vi "DailyReportTry.vi"() -> ()   [LabVIEW 2012]
uses:
  <vilib>/addons/database/Auxilliary.llb/DB Tools Cursor Type.ctl
  <vilib>/addons/database/Connection.llb/DB Tools Open Connec (Path).vi
  <vilib>/addons/database/Connection.llb/Conn Execute.vi
  <vilib>/addons/database/Recordset.llb/Rec Fetch Recordset Data (R).vi
  <vilib>/addons/database/Recordset.llb/Rec Destroy - Connection.vi
  <vilib>/addons/database/_DB Variant To Data/Database Variant To Data.xnode
  <vilib>/addons/database/NI_Database_API.lvlib
panel:
  out "trimmed string":string
  in  "Customer":string(combo)
  in  "error in (no error)":errorcluster
  out "error out":errorcluster
  in  "input cluster":cluster{"String":string, "Value":string}
  in  "connection information":path=path "c:/m100/data/m1003.dsn"
  in  "Device":string(combo)
  out "Boolean":bool
  in  "From Date (起日)":string="2014/9/20"
  in  "離開":bool
  in  "執行":bool
  in  "Shift (班別)":string(combo)
  in  "End Date (ùら)":string="2014/9/24"
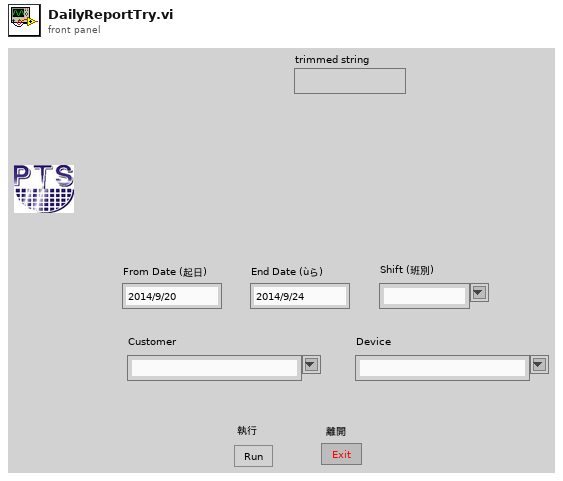
[diagram p1: front panel]
types:
  T1 = typedef "NI_Database_API.lvlib/DB Tools Cursor Type.ctl" = enum16{"forward-only", "keyset", "dynamic", "static"}
  T2 = typedef "NI_Database_API.lvlib/Conn ObjectReference.ctl" = refnum<k1>
  T3 = typedef "NI_Database_API.lvlib/Rec ObjectReference.ctl" = refnum<k1>
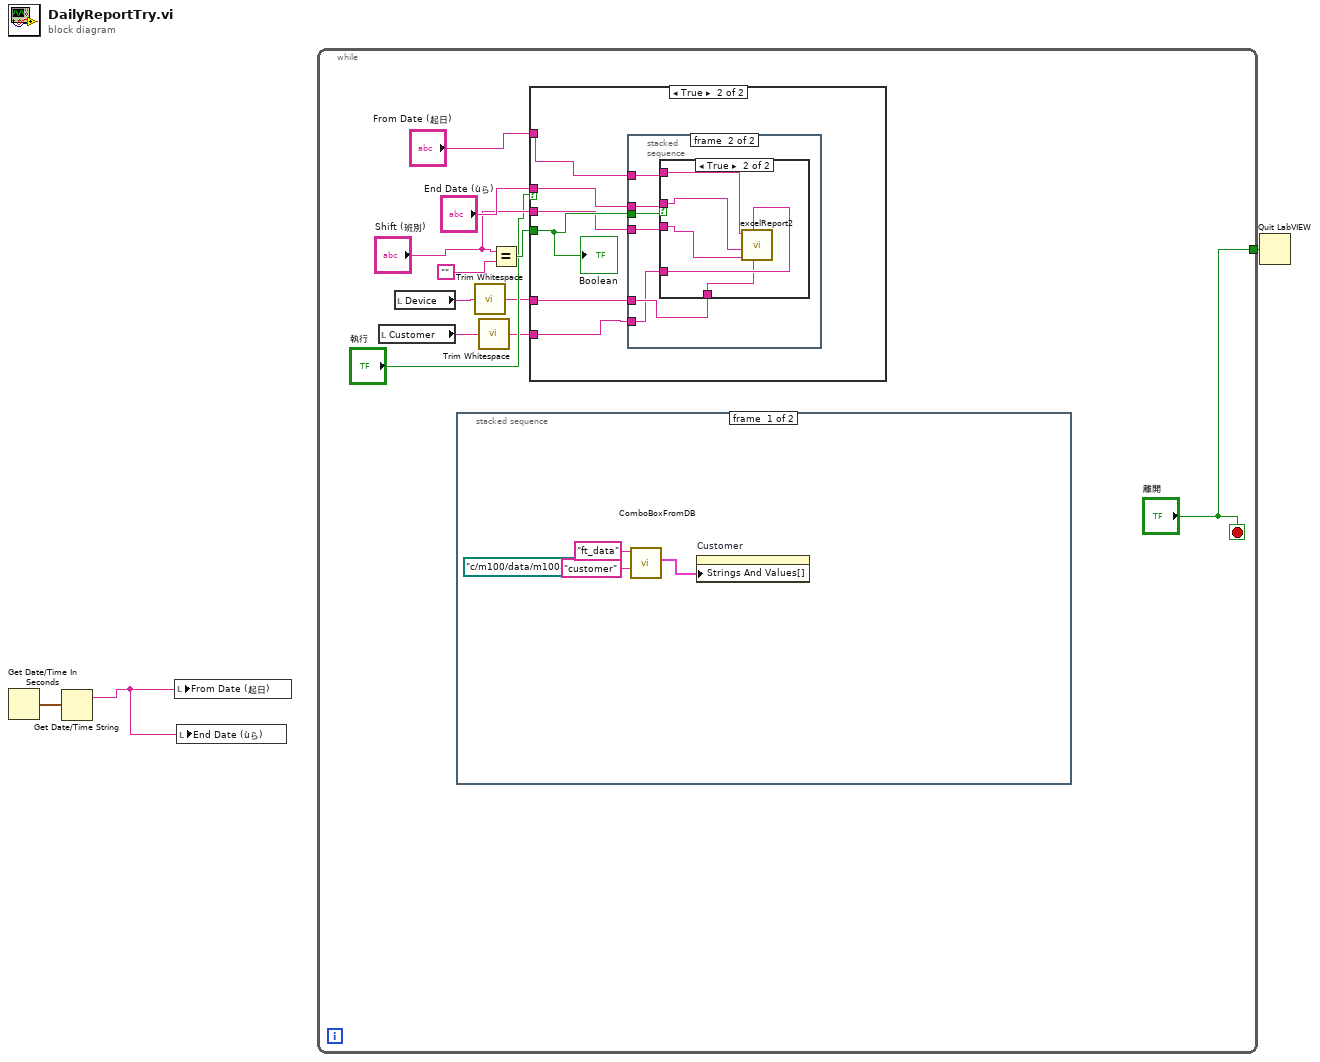
[diagram p0: block diagram]
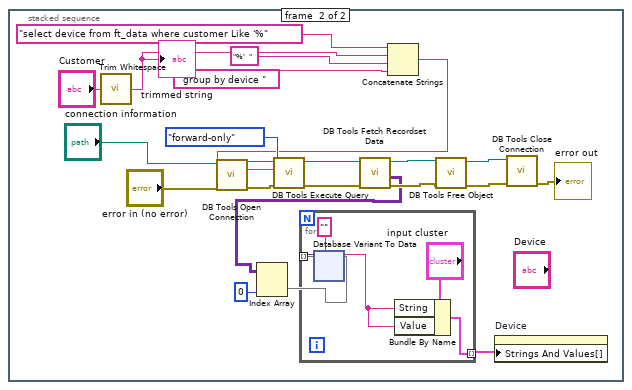
[diagram p2: hidden frame]
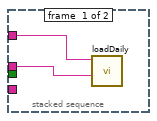
[diagram p4: hidden frame]
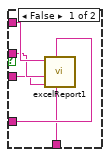
[diagram p5: hidden frame]
diagram:
  n1 = Get Date/Time In Seconds() -> (seconds since 1Jan1904=w1:timestamp)
  n2 = Get Date/Time String(seconds (now)=w1) -> (date string=w2:string)  [unwired: 2 in, 1 out]
  n3 = local write "From Date (起日)"(w2) -> ()
  n4 = local write "End Date (ùら)"(w2) -> ()
  n5 = while {
    tunnel: ["離開"] -> w3
    stop <- "離開" stop-if-true
    n6 = local read "Customer"() -> (w6:string)
    n7 = local read "Device"() -> (w8:string)
    n8 = stacked-sequence {
      frame #0 {
        n9 = call "ComboBoxFromDB.vi"("connection information"=path "c:/m100/data/m1003.dsn", "Column"="customer", "table"="ft_data") -> ("Array"=w15:cluster{"String":string, "Value":string}[])  [unwired: 7 in, 1 out]
        n10 = property on="Customer" class="CmbBox"("Strings And Values[]"=w15) -> ()  [unwired: 2 in, 2 out]
      }
      frame #1 {
        n11 = call <vilib>:"Trim Whitespace.vi"("string"="Customer") -> ("trimmed string"=w19:string)  [unwired: 1 in]
        "trimmed string" <- w19
        n12 = call-poly <vilib>:"DB Tools Open Connection.vi"("error in (no error)"="error in (no error)", "connection information"="connection information") -> ("error out"=w37:errorcluster, "connection reference"=w38:T2)  [unwired: 6 in]
        n13 = Concatenate Strings("select device from ft_data where customer Like '%" ("string"), w19, "%'  " ("string"), " group by device " ("string")) -> (w24:string)
        n14 = call-poly <vilib>:"DB Tools Execute Query.vi"("error in (no error)"=w37, "cursor type"=DB_Tools_Cursor_Type."forward-only", "SQL query"=w24, "connection reference"=w38) -> ("error out"=w32:errorcluster, "recordset reference"=w33:T3)  [unwired: 4 in]
        n15 = call-poly <vilib>:"DB Tools Fetch Recordset Data.vi"("error in (no error)"=w32, "recordset reference"=w33) -> ("error out"=w30:errorcluster, "recordset data"=w29:variant[][], "recordset reference out"=w31:T3)  [unwired: 3 in]
        n16 = Index Array(array=w29, index (col)=0) -> (element=w28:variant[])  [unwired: 1 in]
        n17 = for {
          tunnel: w28 -> [w45] mode=indexing
          tunnel: [w41] -> w21 mode=indexing
          n18 = xnode "Database Variant To Data"("database variant"=w45, "type"="") -> ("data"=w42:string)  [unwired: 1 in, 1 out]
          n19 = Bundle By Name(cluster="input cluster", "String"=w42, "Value"=w42) -> (w41:cluster{"String":string, "Value":string})
        }
        n20 = call-poly <vilib>:"DB Tools Free Object.vi"("error in (no error)"=w30, "recordset reference"=w31) -> ("error out"=w35:errorcluster, "connection reference"=w36:T2)  [unwired: 8 in]
        n21 = property on="Device" class="CmbBox"("Strings And Values[]"=w21) -> ()  [unwired: 2 in, 2 out]
        n22 = call <vilib>:"DB Tools Close Connection.vi"("error in (no error)"=w35, "connection reference"=w36) -> ("error out"=→"error out":errorcluster)  [unwired: 5 in]
      }
    }
    n23 = call <vilib>:"Trim Whitespace.vi"("string"=w8) -> ("trimmed string"=w7:string)  [unwired: 1 in]
    n24 = call <vilib>:"Trim Whitespace.vi"("string"=w6) -> ("trimmed string"=w5:string)  [unwired: 1 in]
    n25 = Equal?(x="Shift (班別)", y="") -> (x = y?=w13:bool)
    n26 = case shown="True" "執行" {
      tunnel: w13 -> [_ w83]
      tunnel: "End Date (ùら)" -> [_ w82]
      tunnel: "Shift (班別)" -> [_ w81]
      tunnel: w7 -> [_ w80]
      tunnel: w5 -> [_ w79]
      tunnel: "From Date (起日)" -> [_ w78]
      frame False {
      }
      frame True {
        n27 = stacked-sequence {
          tunnel: w78 -> [w85 w91]
          tunnel: w83 -> [_ w89]
          tunnel: w82 -> [w84 w90]
          tunnel: w81 -> [_ w88]
          tunnel: w80 -> [_ w87]
          tunnel: w79 -> [_ w86]
          frame #0 {
            n28 = call "loadDaily.vi"("end date"=w84, "begin date"=w85) -> ()  [unwired: 9 in, 1 out]
          }
          frame #1 {
            n29 = case shown="True" w89 {
              tunnel: w91 -> [w96 w101]
              tunnel: w90 -> [w95 w100]
              tunnel: w88 -> [w94 w99]
              tunnel: w86 -> [w93 w98]
              tunnel: w87 -> [w92 w97]
              frame False {
                n30 = call "excelReport1.vi"("device"=w92, "Customer"=w93, "Shift"=w94, "End Date"=w95, "From Date"=w96) -> ()  [unwired: 7 in]
              }
              frame True {
                n31 = call "excelReport2.vi"("device"=w97, "customer"=w98, "Shift"=w99, "End Date"=w100, "From Date"=w101) -> ()  [unwired: 7 in]
              }
            }
          }
        }
        "Boolean" <- w83
      }
    }
  }
  n32 = Quit LabVIEW(quit? (T)=w3) -> ()
